vi "AES ECU Event Measurement - Time Duration.vi"(6 "Cycles to Filter":u16, 10 "Digital Input Pulse":bool) -> (3 "Time Duration (clock ticks)":u32)   [LabVIEW 2010, in "AES.lvlib" / "AES FPGA.lvlib"]
doc: "This IP inputs the fuel injector or ignition coil digital signals from an ECU and determines the Time Duration of the pulses for those signals. A \"Cycles to Filter\" input is also accepted in order to filter the digital inputs for a specified number of SCTL iterations. This is necessary since ECUs often output very noisy signals, and we need to filter it to get accurate calculations on the Start and End Angles."
uses:
  AES FPGA.lvlib
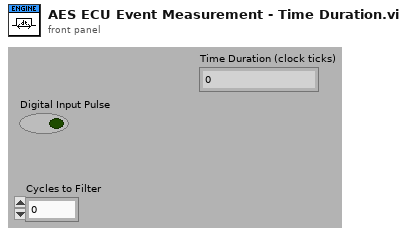
[diagram p1: front panel]
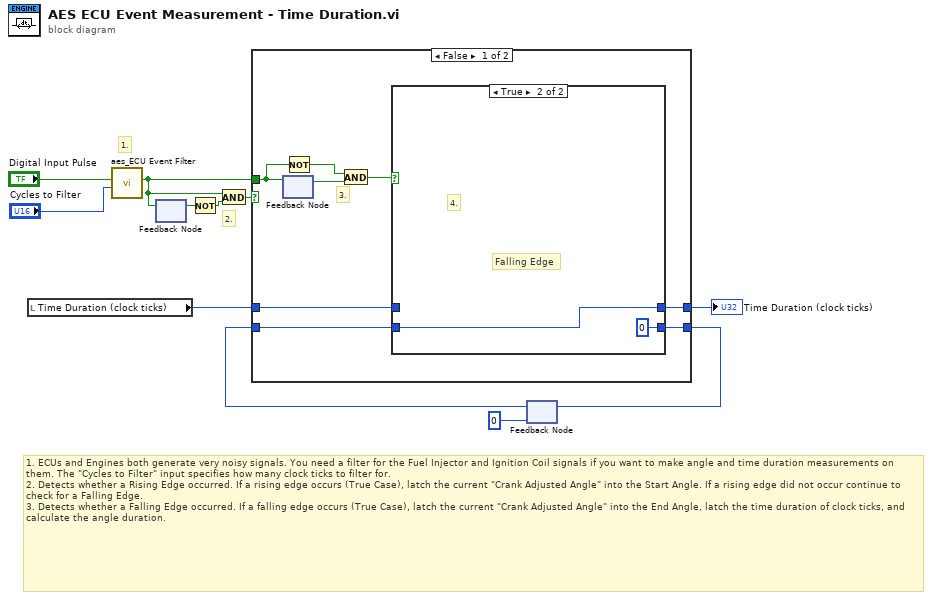
[diagram p0: block diagram]
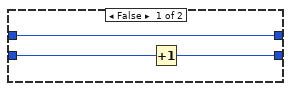
[diagram p2: hidden frame]
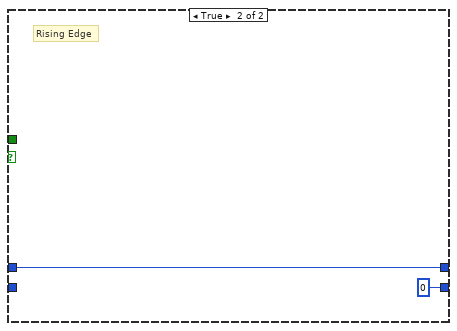
[diagram p3: hidden frame]
diagram:
  # "2."
  # "1. ECUs and Engines both generate very noisy signals. You need a filter for the Fuel Injector and Ignition Coil signals if you want to make angle and time duration measurements on them. The \"Cycles to Filter\" input specifies how many clock ticks to filter for.\n2. Detects whether a Rising Edge occurred. If a rising edge occurs (True Case), latch the current \"Crank Adjusted Angle\" into the Start Angle. If a rising edge did not occur continue to check for a Falling Edge.\n3. Detects whether a Falling Edge occurred. If a falling edge occurs (True Case), latch the current \"Crank Adjusted Angle\" into the End Angle, latch the time duration of clock ticks, and calculate the angle duration."
  # "1."
  n1 = local read "Time Duration (clock ticks)"() -> (w6:u32)
  n2 = call "aes_ECU Event Filter.vi"("Cycles to Filter"="Cycles to Filter", "Input Signal"="Digital Input Pulse") -> ("Output Filtered Signal"=w2:bool)  [unwired: 8 in, 1 out]
  n3 = feedback-in #1(w2) -> ()
  n4 = feedback #1() -> (w11:bool)  [unwired: 1 out]
  n5 = Not(x=w11) -> (.not. x?=w10:bool)
  n6 = And(x=w2, y=w10) -> (x .and. y?=w9:bool)
  n7 = feedback #2(u32 0) -> (w4:u32)
  n8 = case shown="False" w9 {
    tunnel: w2 -> [w16 _]
    tunnel: [w15 w26] -> w8
    tunnel: w6 -> [w14 w26]
    tunnel: [w13 u32 0] -> w5
    tunnel: w4 -> [w12 _]
    frame False {
      # "3."
      n9 = feedback-in #3(w16) -> ()
      n10 = feedback #3() -> (w18:bool)  [unwired: 1 out]
      n11 = Not(x=w16) -> (.not. x?=w17:bool)
      n12 = And(x=w17, y=w18) -> (x .and. y?=w19:bool)
      n13 = case shown="True" w19 {
        tunnel: [w22 w24] -> w15
        tunnel: w14 -> [w22 _]
        tunnel: [w21 u32 0] -> w13
        tunnel: w12 -> [w20 w24]
        frame False {
          n14 = Increment(x=w20) -> (x+1=w21:u32)
        }
        frame True {
          # "4."
          # "Falling Edge"
        }
      }
    }
    frame True {
      # "Rising Edge"
    }
  }
  "Time Duration (clock ticks)" <- w8
  n15 = feedback-in #2(w5) -> ()
